vi "Read piece.vi"(8 "error in (no error)":errorcluster, 10 "Square":T1={"File"=enum."a", "Rank"=enum."4"}, 11 "Board in":refnum<class "Board.lvclass">) -> (0 "error out":errorcluster, 2 "Piece":refnum<class "Piece.lvclass">, 3 "Board out":refnum<class "Board.lvclass">)   [LabVIEW 2016, in "Chesslib.lvlib" / "Board.lvclass"]
uses:
  Board.lvclass
  typedef/Square.ctl
  typedef/File.ctl
  typedef/Rank.ctl
  Pieces/Piece/Piece.lvclass
  Board.lvclass/Board.ctl
  <vilib>/Utility/error.llb/Error Cluster From Error Code.vi
  <vilib>/ErrorRing/Error Ring.xnode
  Chesslib.lvlib
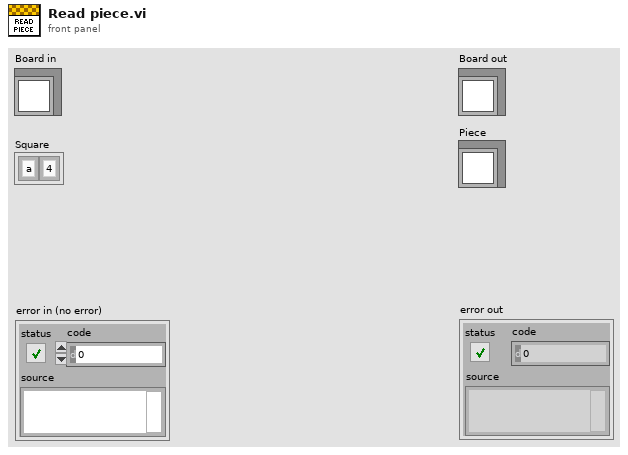
[diagram p1: front panel]
types:
  T1 = typedef "Chesslib.lvlib/Square.ctl" = cluster{"File":T2, "Rank":T3}
  T2 = typedef "Chesslib.lvlib/File.ctl" = enum8{"a", "b", "c", "d", "e", "f", "g", "h"}
  T3 = typedef "Chesslib.lvlib/Rank.ctl" = enum8{"1", "2", "3", "4", "5", "6", "7", "8"}
  T4 = typedef "Chesslib.lvlib/Board.lvclass/Square content.ctl" = cluster{"Occupied":bool, "Piece":refnum<class "Piece.lvclass">}
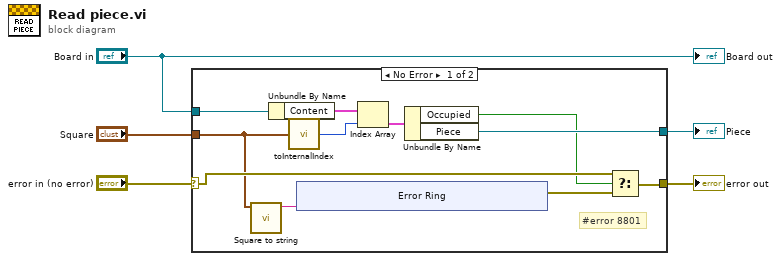
[diagram p0: block diagram]
diagram:
  n1 = case shown="No Error" "error in (no error)" {
    selector: "error in (no error)" -> [w10 w24]
    tunnel: "Square" -> [w6 _]
    tunnel: "Board in" -> [w14 _]
    tunnel: [w12 _] -> w3
    tunnel: [w11 w24] -> w1
    frame No Error {
      # "#error 8801"
      n2 = call "Square to string.vi"("Square"=w6) -> ("Square string"=w7:string)  [unwired: 10 in]
      n3 = Unbundle By Name(w14) -> ("Content"=w15:T4[])
      n4 = call "toInternalIndex.vi"("Square"=w6) -> ("Internal index"=w16:i32)
      n5 = xnode "Error Ring"("parameter 0"=w7) -> ("error out"=w8:errorcluster)
      n6 = Index Array(array=w15, index=w16) -> (element=w13:T4)
      n7 = Unbundle By Name(w13) -> ("Occupied"=w9:bool, "Piece"=w12:refnum<class "Piece.lvclass">)
      n8 = Select(t=w10, s=w9, f=w8) -> (s? t:f=w11:errorcluster)
    }
    frame Error {
    }
  }
  "Piece" <- w3
  "error out" <- w1
  "Board out" <- "Board in"
